vi "Get Wrapper DLL Path.vi"() -> (0 "Wrapper DLL Path":path)   [LabVIEW 2014, in "Keyence LJ-V7000.lvlib"]
uses:
  Keyence LJ-V7000.lvlib
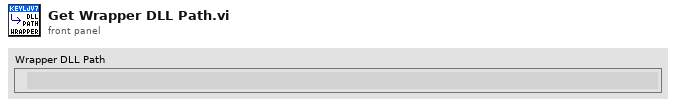
[diagram p1: front panel]
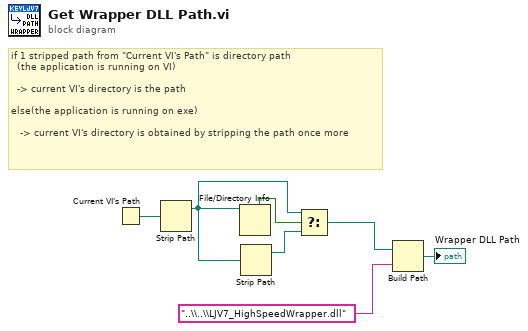
[diagram p0: block diagram]
diagram:
  # "if 1 stripped path from \"Current VI's Path\" is directory path\n  (the application is running on VI)\n\n  -> current VI's directory is the path\n\nelse(the application is running on exe)\n\n　-> current VI's directory is obtained by stripping the path once more"
  n1 = Current VI's Path() -> (path=w3:path)
  n2 = Strip Path(path=w3) -> (stripped path=w2:path)  [unwired: 1 out]
  n3 = File/Directory Info(path=w2) -> (directory=w5:bool)  [unwired: 1 in, 6 out]
  n4 = Strip Path(path=w2) -> (stripped path=w4:path)  [unwired: 1 out]
  n5 = Select(t=w2, s=w5, f=w4) -> (s? t:f=w1:path)
  n6 = Build Path(base path=w1, name or relative path="..\\..\\LJV7_HighSpeedWrapper.dll" ("名前または相対パス")) -> (appended path=→"Wrapper DLL Path":path)
